vi "Read QO2 DVR.vi"(8 "error in (no error)":errorcluster, 11 "Set Rel QO2 flow in":refnum<class "Set Rel QO2 flow.lvclass">) -> (0 "error out":errorcluster, 2 "QO2 DVR":refnum<data-value>, 3 "Set Rel QO2 flow out":refnum<class "Set Rel QO2 flow.lvclass">)   [LabVIEW 2015, in "Set Rel QO2 flow.lvclass"]
uses:
  Set Rel QO2 flow.lvclass
  Set Rel QO2 flow.lvclass/Set Rel QO2 flow.ctl
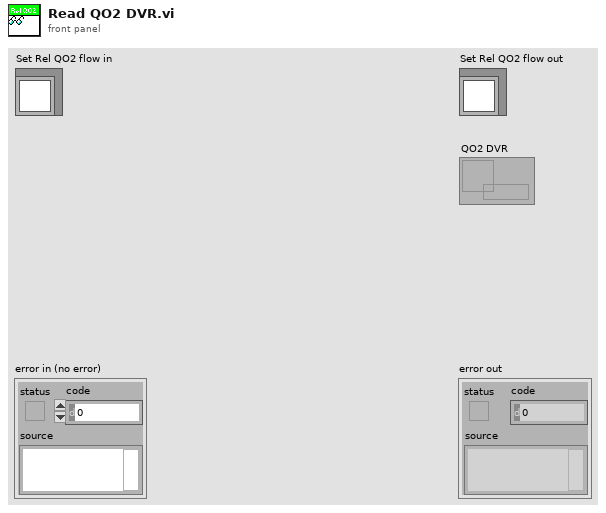
[diagram p1: front panel]
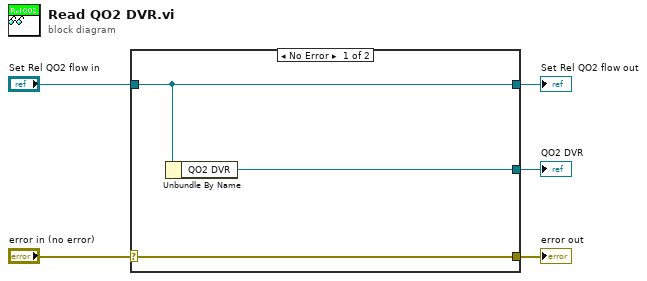
[diagram p0: block diagram]
diagram:
  n1 = case shown="No Error" "error in (no error)" {
    selector: "error in (no error)" -> [w8 w9]
    tunnel: [w8 w9] -> w4
    tunnel: [w7 w10] -> w2
    tunnel: "Set Rel QO2 flow in" -> [w7 w10]
    tunnel: [w6 _] -> w1
    frame No Error {
      n2 = Unbundle By Name(w7) -> ("QO2 DVR"=w6:refnum<data-value>)
    }
    frame Error {
    }
  }
  "error out" <- w4
  "Set Rel QO2 flow out" <- w2
  "QO2 DVR" <- w1
